vi "Measurement Logic.vi"() -> ()   [LabVIEW 2021, in "NIDAQmxMeasurement.lvlib"]
uses:
  NIDAQmxMeasurement.lvlib
  <vilib>/Plug-In SDKs/Measurements/Measure Call Context/Measure Call Context.lvclass
  Measurement Configuration.ctl
  Measurement Results.ctl
  <vilib>/Plug-In SDKs/Clients/Session Management V1/Session Reservation/Initialize and Close Session Behavior.ctl
  <vilib>/Plug-In SDKs/Measurements/Measure Call Context/Reserve Sessions - 1Pin.vi
  <vilib>/Plug-In SDKs/Sessions/niDAQmx/Initialize Tasks - 1Task.vi
  <vilib>/Plug-In SDKs/Sessions/niDAQmx/Get Connections - 1Pin 1Conn.vi
  <vilib>/Plug-In SDKs/Sessions/niDAQmx/Session Management niDAQmx.lvlib
  <vilib>/Plug-In SDKs/Clients/Session Management V1/Session Reservation/Session Reservation.lvclass
panel:
  out "measurement results":T1
  in  "measurement configuration":T2
  out "measure call context out":refnum<class "Measure Call Context.lvclass">
  in  "measure call context in":refnum<class "Measure Call Context.lvclass">
  out "error out":errorcluster
  in  "error in":errorcluster
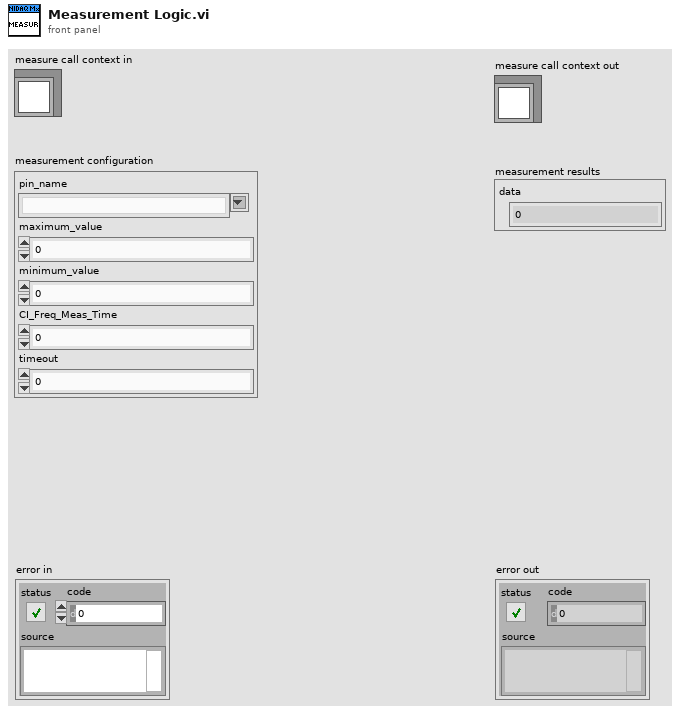
[diagram p1: front panel]
types:
  T1 = typedef "NIDAQmxMeasurement.lvlib/Measurement Results.ctl" = cluster{"data":dbl}
  T2 = typedef "NIDAQmxMeasurement.lvlib/Measurement Configuration.ctl" = cluster{"pin_name":string, "maximum_value":dbl, "minimum_value":dbl, "CI_Freq_Meas_Time":dbl, "timeout":dbl}
  T3 = typedef "NI Session Management V1 Client.lvlib/Session Reservation.lvclass/Initialize and Close Session Behavior.ctl" = enum16{"Auto", "Initialize and Close", "Attach and Detach", "Initialize and Detach", "Attach and Close"}
  T4 = typedef "Session Management niDAQmx.lvlib/Connection with Session.ctl" = cluster{"connection":T5, "session":refnum<class "Session Factory.lvclass">}
  T5 = typedef "NI Session Management V1 Client.lvlib/Session Reservation.lvclass/Connection.ctl" = cluster{"pin or relay name":string, "site":i32, "instrument type id":string, "channel":string}
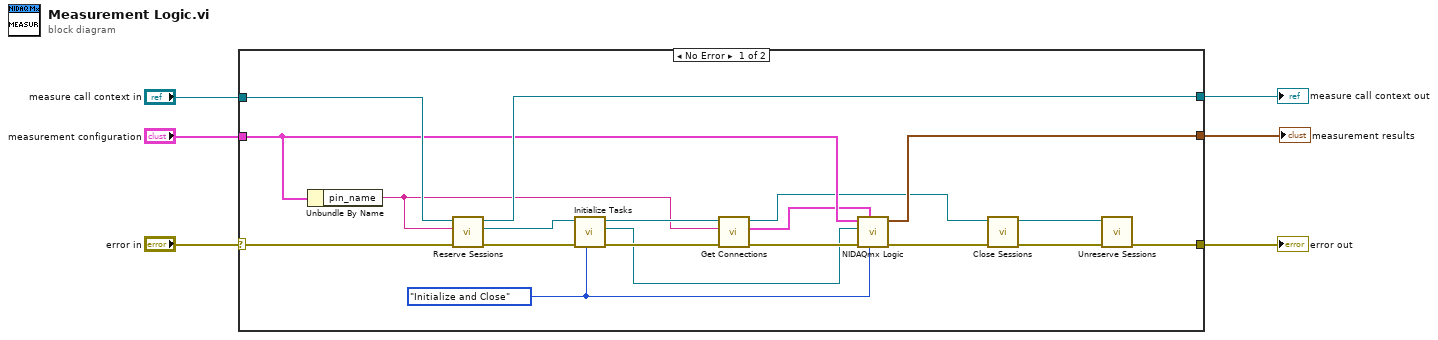
[diagram p0: block diagram]
diagram:
  n1 = case shown="No Error" "error in" {
    selector: "error in" -> [w23 w26]
    tunnel: "measure call context in" -> [w25 w27]
    tunnel: [w24 w27] -> w5
    tunnel: [w20 w26] -> w3
    tunnel: "measurement configuration" -> [w17 _]
    tunnel: [w18 _] -> w1
    frame No Error {
      w7 = Initialize_and_Close_Session_Behavior."Initialize and Close" ("initialize and close session behavior")
      n2 = Unbundle By Name(w17) -> ("pin_name"=w11:string)
      n3 = call-poly <vilib>:"Reserve Sessions.vi"("error in"=w23, "pin or relay name"=w11, "measurement context in"=w25) -> ("error out"=w16:errorcluster, "session reservation out"=w15:refnum<class "Session Reservation.lvclass">, "measurement context out"=w24:refnum<class "Measure Call Context.lvclass">)  [unwired: 6 in]
      n4 = call-poly <vilib>:"Initialize Tasks.vi"("initialize and close session behavior"=w7, "error in"=w16, "session reservation in"=w15) -> ("error out"=w14:errorcluster, "task"=w8:refnum<class "Session Factory.lvclass">, "session reservation out"=w12:refnum<class "Session Reservation.lvclass">)  [unwired: 5 in, 1 out]
      n5 = call-poly <vilib>:"Get Connections.vi"("error in"=w14, "pin or relay name"=w11, "session reservation in"=w12) -> ("error out"=w13:errorcluster, "connection"=w10:T4, "session reservation out"=w9:refnum<class "Session Reservation.lvclass">)  [unwired: 6 in]
      n6 = call "NIDAQmx Logic.vi"("initialize and close session behavior"=w7, "connection type"=w10, "error in (no error)"=w13, "Session Factory in"=w8, "Measurement Configuration"=w17) -> ("error out"=w22:errorcluster, "Measurement Results"=w18:T1)  [unwired: 5 in]
      n7 = call <vilib>:"Close Sessions.vi"("error in"=w22, "session reservation in"=w9) -> ("error out"=w21:errorcluster, "session reservation out"=w19:refnum<class "Session Reservation.lvclass">)  [unwired: 8 in]
      n8 = call <vilib>:"Unreserve Sessions.vi"("error in"=w21, "session reservation in"=w19) -> ("error out"=w20:errorcluster)  [unwired: 9 in]
    }
    frame Error {
    }
  }
  "error out" <- w3
  "measure call context out" <- w5
  "measurement results" <- w1
